vi "Broadcast-status.vi"(8 "error in (no error)":errorcluster, 10 "Status":T1, 11 "Client in":T2) -> (0 "error out":errorcluster, 3 "Client out":T2)   [LabVIEW 2013, in "PowderDeposition.lvlib" / "PD-Client.lvclass"]
doc: "Wrapper function for sending the specific 'Hearbeat' type message.\nThis function creates and immediately sends a heartbeat message to the server, using the configuration of the client object."
uses:
  PD-Client.lvclass
  Object-reference.ctl
  Main/Client-status.ctl
  SA-SLMAPI/Sources/Send-status/Send-status.lvclass
  Main/PD-Main.lvclass
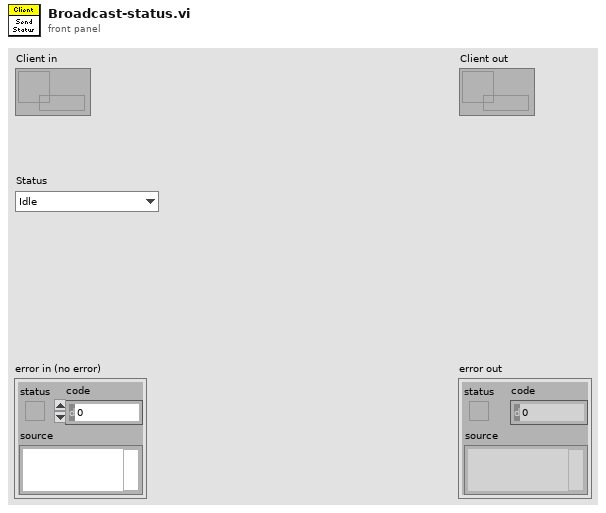
[diagram p1: front panel]
types:
  T1 = typedef "PowderDeposition.lvlib/PD-Main.lvclass/Client-status.ctl" = enum16{"Idle", "Initialized", "Configured", "Activated", "Started", "Paused", "Stopped", "Reset", "Error", "Exited"}
  T2 = typedef "PowderDeposition.lvlib/PD-Client.lvclass/Object-reference.ctl" = refnum<data-value>
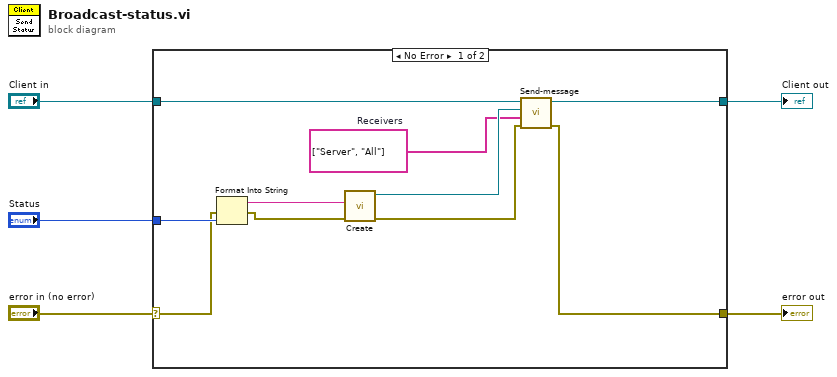
[diagram p0: block diagram]
diagram:
  n1 = case shown="No Error" "error in (no error)" {
    selector: "error in (no error)" -> [w13 w17]
    tunnel: "Client in" -> [w10 w16]
    tunnel: [w15 w16] -> w4
    tunnel: [w7 w17] -> w2
    tunnel: "Status" -> [w14 _]
    frame No Error {
      w6 = string[] ["Server", "All"]  # Receivers
      n2 = Format Into String(error in=w13, w14) -> (resulting string=w12:string, error out=w8:errorcluster)  [unwired: 2 in]
      n3 = call "Create.vi"("error in (no error)"=w8, "Status"=w12) -> ("error out"=w9:errorcluster, "Send-status out"=w11:refnum<class "Send-status.lvclass">)  [unwired: 8 in]
      n4 = call "Send-message.vi"("error in (no error)"=w9, "Receivers"=w6, "Message"=w11, "Client in"=w10) -> ("error out"=w7:errorcluster, "Client out"=w15:T2)  [unwired: 6 in]
    }
    frame Error {
    }
  }
  "error out" <- w2
  "Client out" <- w4
